vi "RegisterDataSets.vi"(8 "error in (no error)":errorcluster, 10 "RegisterDataSet":T1, 11 "registry in":variant) -> (0 "error out":errorcluster, 3 "registry out":variant)   [LabVIEW 2017, in "DataEventCreator.lvlib"]
uses:
  <vilib>/addons/InsightCM/Devices/Shared/Common/DataEventCreator/controls/RegisterDataSets.ctl
  <vilib>/addons/InsightCM/Devices/Shared/Cms/CmsDataEventCreator/controls/DataSetRegistry.ctl
  <vilib>/addons/InsightCM/Devices/Shared/Common/DataEvent/controls/DataSetType.ctl
  <vilib>/addons/InsightCM/Devices/Shared/Cms/CmsDataEventCreator/controls/GroupRegistry.ctl
  <vilib>/addons/InsightCM/Devices/Shared/Common/DataEventCreator/controls/Registry_Trend.ctl
  <vilib>/addons/InsightCM/Devices/Shared/Common/DataEventCreator/DataEventCreator.lvlib
  <vilib>/addons/InsightCM/Devices/Shared/Common/DataEvent/DataEvent.lvlib
  <vilib>/addons/InsightCM/Devices/Shared/Cms/CmsDataEventCreator/CmsDataEventCreator.lvlib
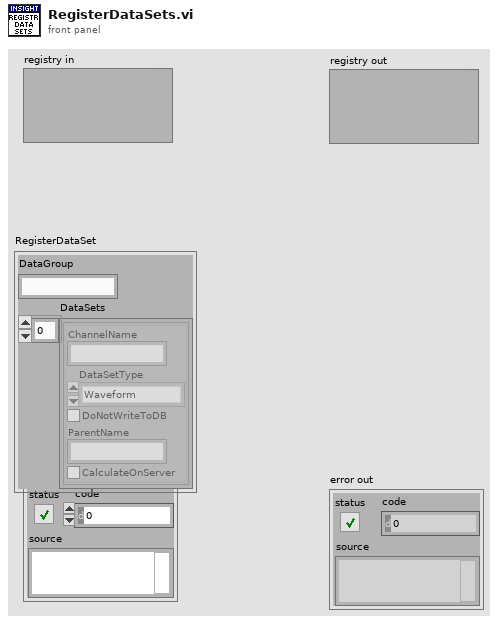
[diagram p1: front panel]
types:
  T1 = typedef "DataEventCreator.lvlib/RegisterDataSets.ctl" = cluster{"DataGroup":string, "DataSets":T2[]}
  T2 = typedef "CmsDataEventCreator.lvlib/DataSetRegistry.ctl" = cluster{"ChannelName":string, "DataSetType":T3, "DoNotWriteToDB":bool, "ParentName":string, "CalculateOnServer":bool}
  T3 = typedef "DataEvent.lvlib/DataSetType.ctl" = enum16{"Waveform", "SpeedProfile", "ThermalImage", "EmsaSweep"}
  T4 = typedef "CmsDataEventCreator.lvlib/GroupRegistry.ctl" = cluster{"AssetNodeMap":variant, "DataSets":T2[], "Trends":T5[]}
  T5 = typedef "DataEventCreator.lvlib/Registry_Trend.ctl" = cluster{"TrendPointId":string, "DataSetName":string, "HighRate":bool, "Always Send":bool}
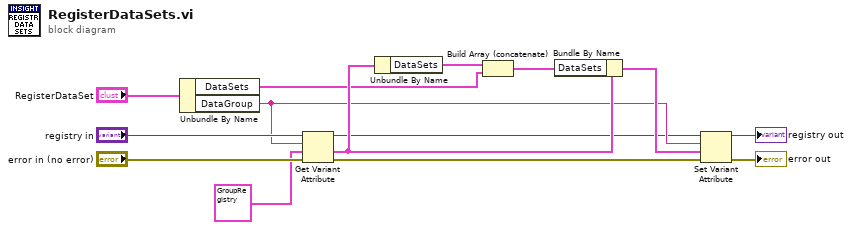
[diagram p0: block diagram]
diagram:
  n1 = Unbundle By Name("RegisterDataSet") -> ("DataSets"=w1:T2[], "DataGroup"=w8:string)
  n2 = Get Variant Attribute(Variant="registry in", name=w8, default value (empty Variant)=T4 {"AssetNodeMap"=variant, "DataSets"=[], "Trends"=[]} ("Data Group Registry"), error in="error in (no error)") -> (duplicate Variant=w4:variant, value=w11:T4, error out=w5:errorcluster)  [unwired: 1 out]
  n3 = Unbundle By Name(w11) -> ("DataSets"=w14:T2[])
  n4 = Build Array (concatenate)(w14, w1) -> (w10:T2[])
  n5 = Bundle By Name(cluster=w11, "DataSets"=w10) -> (w9:T4)
  n6 = Set Variant Attribute(Variant=w4, name=w8, value=w9, error in=w5) -> (Variant out=→"registry out":variant, error out=→"error out":errorcluster)  [unwired: 1 out]
